vi "Create.vi"(8 "error in (no error)":errorcluster, 10 "Input":string) -> (0 "error out":errorcluster, 3 "Measurement":refnum<class "Measurement.lvclass">)   [LabVIEW 2020, in "Measurement.lvclass"]
uses:
  Measurement.lvclass
  Measurement.lvclass/Measurement.ctl
  Helpers/Helpers.lvlib
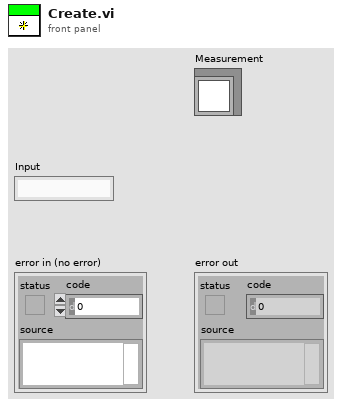
[diagram p1: front panel]
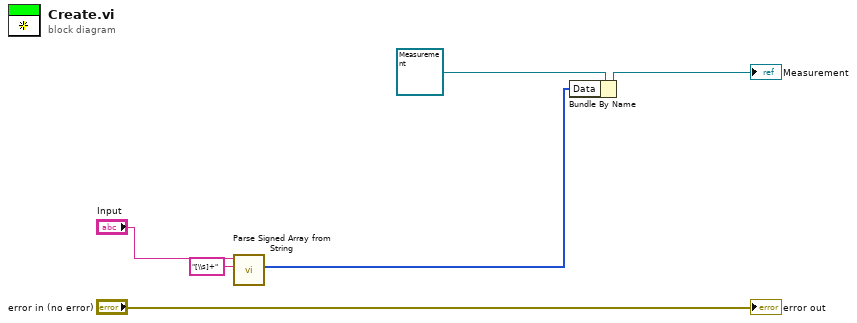
[diagram p0: block diagram]
diagram:
  n1 = call "Parse Signed Array from String.vi"("Delimiter regex"="[\\s]+", "Input"="Input") -> ("Parsed I64 Array"=w1:i64[])  [unwired: 8 in, 1 out]
  n2 = Bundle By Name(cluster=refnum<class "Measurement.lvclass"> refnum ("Measurement"), "Data"=w1) -> (→"Measurement":refnum<class "Measurement.lvclass">)
  "error out" <- "error in (no error)"
